vi "ExTestAdvDispScaling.vi"() -> ()   [LabVIEW 2010]
panel:
  in  "Set Min-Max":bool
  in  "stop":bool
  in  "Set Auto":bool
  in  "Set Manual":bool
  in  "Max":u32=65535
  in  "Min":u32
  in  "Full File Name":path
  out "error out":errorcluster
  in  "error in (no error)":errorcluster
  in  "SITKFULLDISPLAYLib.SITKFullDisplay":refnum<k7>(container)
  # "Browse match pattern is set to *.tif.  Modify this if different file type is needed."
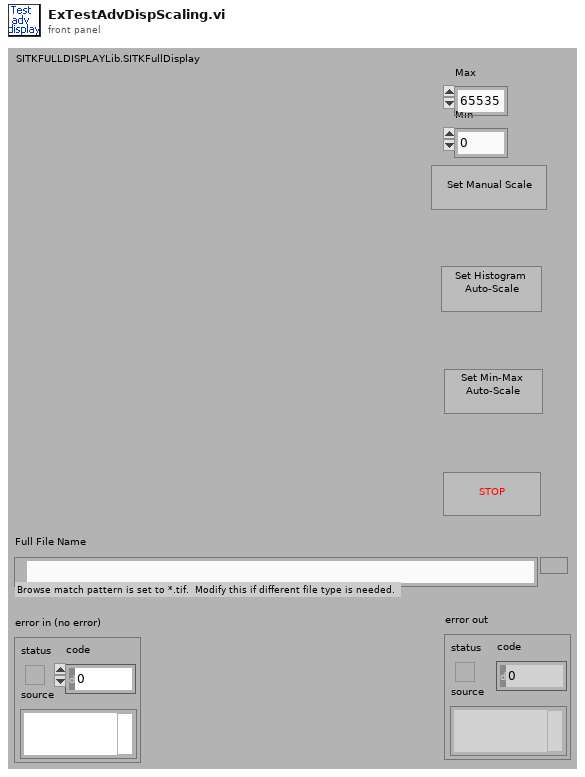
[diagram p1: front panel]
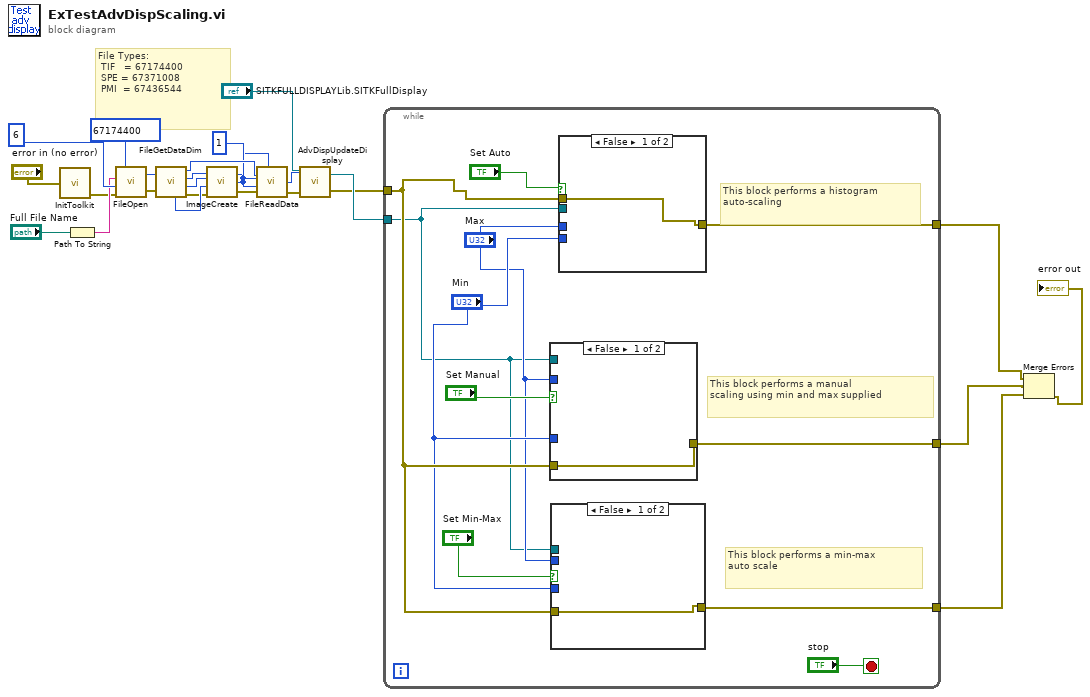
[diagram p0: block diagram]
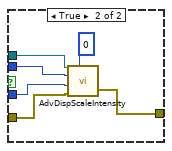
[diagram p2: hidden frame]
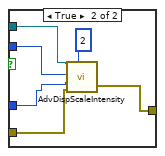
[diagram p3: hidden frame]
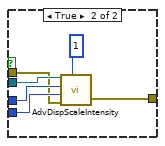
[diagram p4: hidden frame]
diagram:
  w14 = 1
  # "File Types:\n TIF   = 67174400\n SPE = 67371008\n PMI  = 67436544"
  n1 = call <userlib>:"InitToolkit.vi"("error in"="error in (no error)") -> ("error out"=w10:errorcluster)
  n2 = Path To String(path="Full File Name") -> (string=w22:string)
  n3 = call <userlib>:"FileOpen.vi"("error in"=w10, "File Operations"=6, "FileName"=w22, "File Type"=67174400) -> ("error out"=w21:errorcluster, "File Handle"=w20:u32)
  n4 = call <userlib>:"FileGetDataDim.vi"("File Handle"=w20, "error in"=w21) -> ("Data Type"=w17:u32, "File Handle"=w15:u32, "X dim"=w19:u32, "Y dim"=w18:u32, "error out"=w16:errorcluster)  [unwired: 1 out]
  n5 = call <userlib>:"ImageCreate.vi"("X dimension"=w19, "Y dimension"=w18, "Data Type"=w17, "error in"=w16, "Number Of Frames"=w14) -> ("Image Handle"=w12:u32, "error out"=w13:errorcluster)
  n6 = call <userlib>:"FileReadData.vi"("File Handle"=w15, "Start Frame"=w14, "End Frame"=w14, "error in"=w13, "Image Handle"=w12) -> ("Image Handle"=w8:u32, "error out"=w7:errorcluster)  [unwired: 1 out]
  n7 = call <userlib>:"AdvDispUpdateDisplay.vi"("error in (no error)"=w7, "Image Handle"=w8, "SITKFULLDISPLAYLib.SITKFullDisplay"="SITKFULLDISPLAYLib.SITKFullDisplay") -> ("error out"=w5:errorcluster, "SITKFULLDISPLAYLib.SITKFullDisplay"=w6:refnum<k7>)  [unwired: 1 in]
  n8 = while {
    tunnel: w6 -> [w30]
    tunnel: w5 -> [w33]
    tunnel: [w28] -> w3
    tunnel: [w27] -> w2
    tunnel: [w26] -> w1
    stop <- "stop" stop-if-true
    # "This block performs a min-max\nauto scale"
    # "This block performs a histogram\nauto-scaling"
    # "This block performs a manual\nscaling using min and max supplied"
    n9 = case shown="False" "Set Manual" {
      tunnel: w30 -> [_ w50]
      tunnel: "Max" -> [_ w49]
      tunnel: "Min" -> [_ w48]
      tunnel: w33 -> [w44 w47]
      tunnel: [w44 w45] -> w27
      frame False {
      }
      frame True {
        n10 = call <userlib>:"AdvDispScaleIntensity.vi"("SITKFULLDISPLAYLib.SITKFullDisplay"=w50, "High Intensity"=w49, "Low Intensity"=w48, "error in (no error)"=w47, "Type of Scale"=2) -> ("error out"=w45:errorcluster)  [unwired: 1 out]
      }
    }
    n11 = case shown="False" "Set Min-Max" {
      tunnel: w33 -> [w37 w43]
      tunnel: "Min" -> [_ w42]
      tunnel: "Max" -> [_ w41]
      tunnel: w30 -> [_ w40]
      tunnel: [w37 w38] -> w26
      frame False {
      }
      frame True {
        n12 = call <userlib>:"AdvDispScaleIntensity.vi"("SITKFULLDISPLAYLib.SITKFullDisplay"=w40, "High Intensity"=w41, "Low Intensity"=w42, "error in (no error)"=w43, "Type of Scale"=0) -> ("error out"=w38:errorcluster)  [unwired: 1 out]
      }
    }
    n13 = case shown="False" "Set Auto" {
      tunnel: w30 -> [_ w56]
      tunnel: "Max" -> [_ w55]
      tunnel: "Min" -> [_ w54]
      tunnel: w33 -> [w51 w53]
      tunnel: [w51 w52] -> w28
      frame False {
      }
      frame True {
        n14 = call <userlib>:"AdvDispScaleIntensity.vi"("SITKFULLDISPLAYLib.SITKFullDisplay"=w56, "High Intensity"=w55, "Low Intensity"=w54, "error in (no error)"=w53, "Type of Scale"=1) -> ("error out"=w52:errorcluster)  [unwired: 1 out]
      }
    }
  }
  n15 = Merge Errors(w3, w2, w1) -> (→"error out":errorcluster)
